vi "Get Library Path.vi"() -> (0 "Path":path)   [LabVIEW 2020]
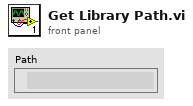
[diagram p1: front panel]
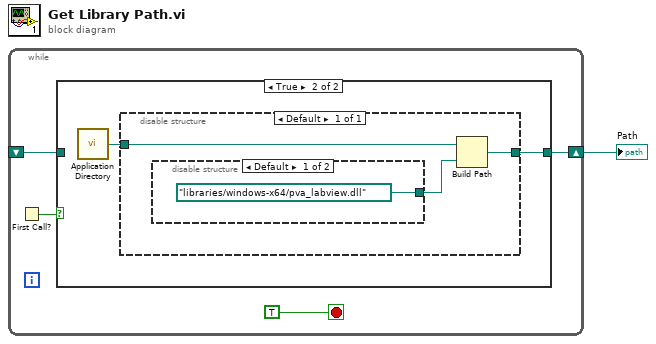
[diagram p0: block diagram]
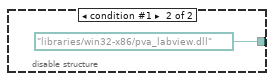
[diagram p3: hidden frame]
diagram:
  n1 = while {
    shift-right: [w5] -> w1
    shift-left: _ -> [w3]
    stop <- TRUE stop-if-true
    n2 = First Call?() -> (First Call?: T/F=w2:bool)
    n3 = case shown="True" w2 {
      tunnel: [w6 w8] -> w5
      tunnel: w3 -> [w6 _]
      frame False {
      }
      frame True {
        n4 = call <vilib>:"Application Directory.vi"() -> ("Application Directory"=w7:path)
        n5 = disable-structure shown="Default" {
          disable-tunnel: w7 -> [w9]
          disable-tunnel: [w11] -> w8
          frame Enabled {
            n6 = disable-structure shown="Default" {
              disable-tunnel: [path "libraries/windows-x64/pva_labview.dll" ("Path") path "libraries/win32-x86/pva_labview.dll" ("Path")] -> w10
              frame condition #0 (active) {
              }
              frame condition #1 {
              }
            }
            n7 = Build Path(base path=w9, name or relative path=w10) -> (appended path=w11:path)
          }
        }
      }
    }
  }
  "Path" <- w1
